vi "CSMSVMgr Initialize.vi"(8 "Error in":errorcluster caption="Error in (no error)") -> (0 "Error out":errorcluster, 3 "INI-Static-Variable-Support.lvlib:CSM-Static-Variable-Manager.lvclass":refnum<class "CSM-Static-Variable-Manager.lvclass">)   [LabVIEW 2017, in "INI-Static-Variable-Support.lvlib" / "CSM-Static-Variable-Manager.lvclass"]
uses:
  CSM-Static-Variable-Manager.lvclass
  INI-Static-Variable-Support.lvlib
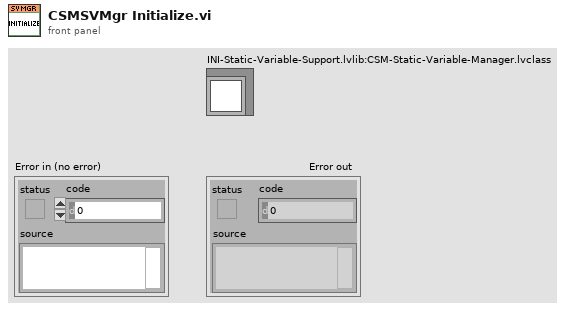
[diagram p1: front panel]
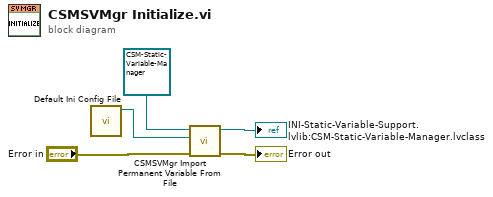
[diagram p0: block diagram]
diagram:
  n1 = call "Default Ini Config File.vi"() -> ("appended path"=w1:path)  [unwired: 11 in]
  n2 = call "CSMSVMgr Import Permanent Variable From File.vi"("error in (no error)"="Error in", "Path"=w1, "CSM-Static-Variable-Manager in"=refnum<class "CSM-Static-Variable-Manager.lvclass"> refnum ("INI-Static-Variable-Support.lvlib:CSM-Static-Variable-Manager.lvclass")) -> ("error out"=→"Error out":errorcluster, "CSM-Static-Variable-Manager out"=→"INI-Static-Variable-Support.lvlib:CSM-Static-Variable-Manager.lvclass":refnum<class "CSM-Static-Variable-Manager.lvclass">)  [unwired: 7 in]
